vi "Global Values.vi"() -> ()   [LabVIEW 2017, in "Simulator Display.xctl"]
uses:
  <vilib>/robotics/Controls/Simulator Display/Simulator Display.xctl
panel:
  in  "MTX Sensor Display":string="Display Sensor Data"
  in  "MTX ID Display":string="Display Robot ID"
  in  "MTX Service":string[](array[string])=["Pause Simulator Service", "Reset Simulator Service"]
  in  "MTX Draw Mode Options":string[](array[string])=["Visual Model Only", "Physics Model Only", "Both"]
  in  "MTX BG Color":string="Background Color"
  in  "MTX Contact Display":string="Draw Contacts"
  in  "MTX Draw Mode":string="Draw Mode"
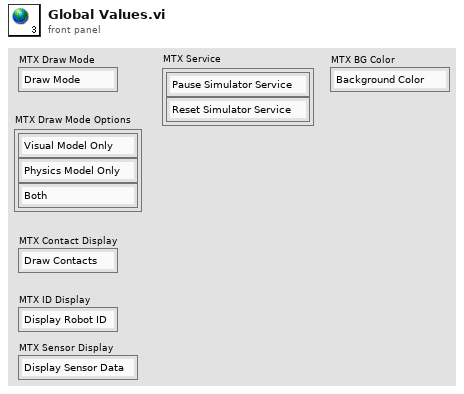
[diagram p1: front panel]
diagram:
